vi "Get Bucket Request Payment.vi"(8 "error in (no error)":errorcluster, 11 "Bucket in":refnum<class "Bucket.lvclass">) -> (0 "error out":errorcluster, 2 "Payer":T1, 3 "Bucket out":refnum<class "Bucket.lvclass">)   [LabVIEW 2015, in "NI_AWS_S3.lvlib" / "Bucket.lvclass"]
doc: "This implementation of the GET operation uses the requestPayment subresource to return the request payment configuration of a bucket. To use this version of the operation, you must be the bucket owner."
uses:
  Bucket.lvclass
  Payer.ctl
  Core/HTTP Request/Region handling.ctl
  Core/HTTP Request/Request Options.ctl
  Core/HTTP Request/Name Value Pair.ctl
  Core/HTTP Request/URL formatting.ctl
  Bucket.lvclass/Bucket.ctl
  Read Name.vi
  Core/HTTP Request/HTTP Request.lvclass
  XML Parsing/NI_XML Parsing.lvlib
  NI_AWS_S3.lvlib
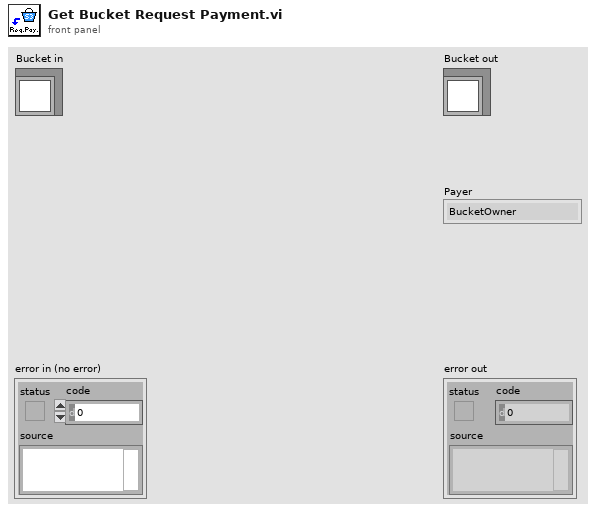
[diagram p1: front panel]
types:
  T1 = typedef "NI_AWS_S3.lvlib/Payer.ctl" = enum16{"BucketOwner", "Requester"}
  T2 = typedef "NI_AWS_Core.lvlib/HTTP Request.lvclass/Name Value Pair.ctl" = cluster{"name":string, "value":string}
  T3 = typedef "NI_AWS_Core.lvlib/HTTP Request.lvclass/Request Options.ctl" = cluster{"request headers":T2[], "request parameters":T2[], "request body":string, "region handling":T4, "URL formatting":T5}
  T4 = typedef "NI_AWS_Core.lvlib/HTTP Request.lvclass/Region handling.ctl" = enum16{"use region everywhere", "use region (authentication only)", "use region (URL only)", "ignore region everwhere"}
  T5 = typedef "NI_AWS_Core.lvlib/HTTP Request.lvclass/URL formatting.ctl" = enum16{"region-", "region."}
  T6 = typedef "NI_AWS_Core.lvlib/HTTP Request.lvclass/Response.ctl" = cluster{"Headers":string, "Body":string}
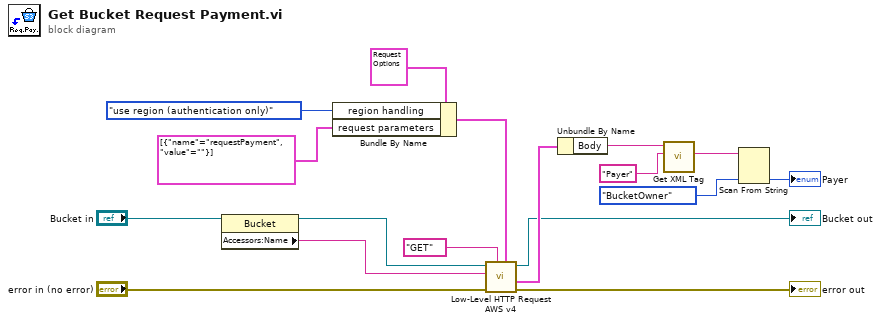
[diagram p0: block diagram]
diagram:
  n1 = property class="Bucket"(reference="Bucket in") -> (reference out=w5:refnum<class "Bucket.lvclass">, "Accessors:Name"=w17:string)  [unwired: 1 in, 1 out]
  n2 = Bundle By Name(cluster=T3 {"request headers"=[], "request parameters"=[], "request body"="", "region handling"=enum."use region everywhere", "URL formatting"=enum."region."} ("Request Options"), "region handling"=Region_handling."use region (authentication only)", "request parameters"=T2[] [{"name"="requestPayment", "value"=""}]) -> (w6:T3)
  n3 = call "Low-Level HTTP Request AWS v4.vi"("Request Options"=w6, "HTTP-Verb"="GET", "error in (no error)"="error in (no error)", "URL Prefix"=w17, "AWS Core in"=w5) -> ("error out"=→"error out":errorcluster, "Response"=w8:T6, "AWS Core out"=→"Bucket out":refnum<class "Bucket.lvclass">)  [unwired: 3 in, 1 out]
  n4 = Unbundle By Name(w8) -> ("Body"=w10:string)
  n5 = call "Get XML Tag.vi"("Tag name"="Payer", "XML String in"=w10) -> ("Tag value"=w3:string)  [unwired: 5 in, 4 out]
  n6 = Scan From String(input string=w3, default 1=Payer."BucketOwner" ("Payer")) -> (output 1=→"Payer":T1)  [unwired: 3 in, 3 out]
